vi "Power Qualtiy - 4.vi"() -> ()   [LabVIEW 2015]
uses:
  <vilib>/addons/Electrical Power/Basic/Measurement/subVIs/basic_Power Value.ctl
  <vilib>/express/express signal manip/GetorSetDDTAttributes/Shared VIs/TimeType.ctl
  <vilib>/express/express signal manip/GetorSetDDTAttributes/Shared VIs/XDimension.ctl
  <vilib>/addons/Electrical Power/Basic/Measurement/RMS (N Channels).vi
  <vilib>/addons/Electrical Power/Basic/Measurement/Power (1 Channel).vi
  <vilib>/express/express signal manip/GetorSetDDTAttributes/Shared VIs/TimeMode Enum to Boolean.vi
  <vilib>/express/express signal manip/GetorSetDDTAttributes/Shared VIs/XDimension Enum to String.vi
  <vilib>/express/express shared/transition.llb/Dynamic To Waveform Array.vi
  <vilib>/express/express signal manip/GetorSetDDTAttributes/Set DDT Attributes/SetT0.vi
  <vilib>/express/express signal manip/GetorSetDDTAttributes/Set DDT Attributes/sub Set StartTimeStamp.vi
  <vilib>/express/express shared/transition.llb/Waveform Array To Dynamic.vi
  <vilib>/express/express signal manip/GetorSetDDTAttributes/Set DDT Attributes/Set DDT Properties.xnode
  <vilib>/express/express signal manip/GetorSetDDTAttributes/Shared VIs/GetSetShared.lvlib
  <vilib>/addons/Electrical Power/Basic/NI_EP_Basic.lvlib
  <vilib>/express/express signal manip/GetorSetDDTAttributes/Set DDT Attributes/Set DDT Attributes.lvlib
panel:
  out "Voltage":dbl(knob) scale=0.0..230.0
  out "power value":T1
  out "Voltage Waveform":dynamicdata(graph)
  out "Current Waveform":dynamicdata(graph)
  out "Current":dbl(knob) scale=0.0..12.0
  out "THD":dbl
  out "Current Harmonics":dynamicdata(graph)
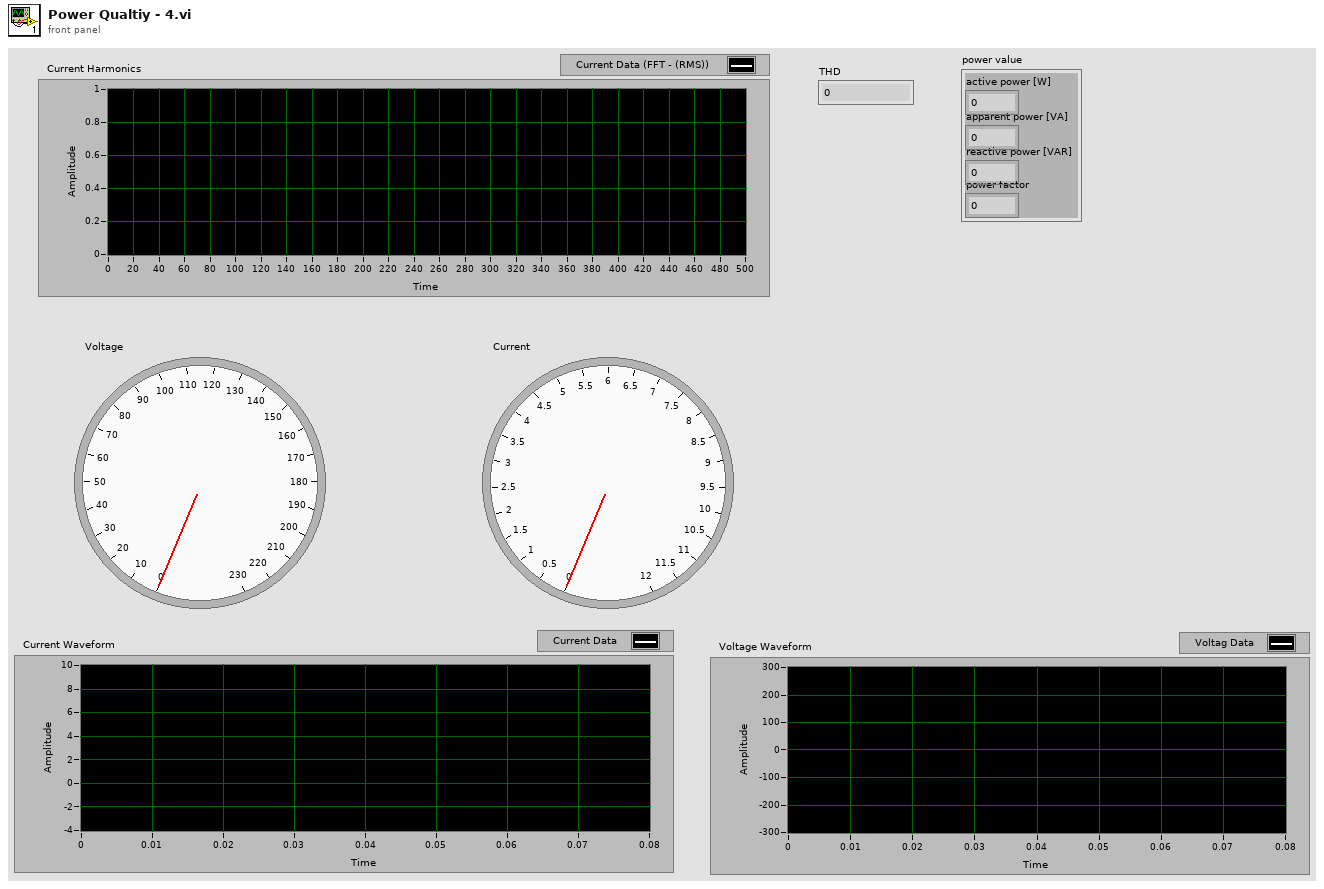
[diagram p1: front panel]
types:
  T1 = typedef "NI_EP_Basic.lvlib/basic_Power Value.ctl" = cluster{"active power [W]":dbl, "apparent power [VA]":dbl, "reactive power [VAR]":dbl, "power factor":dbl}
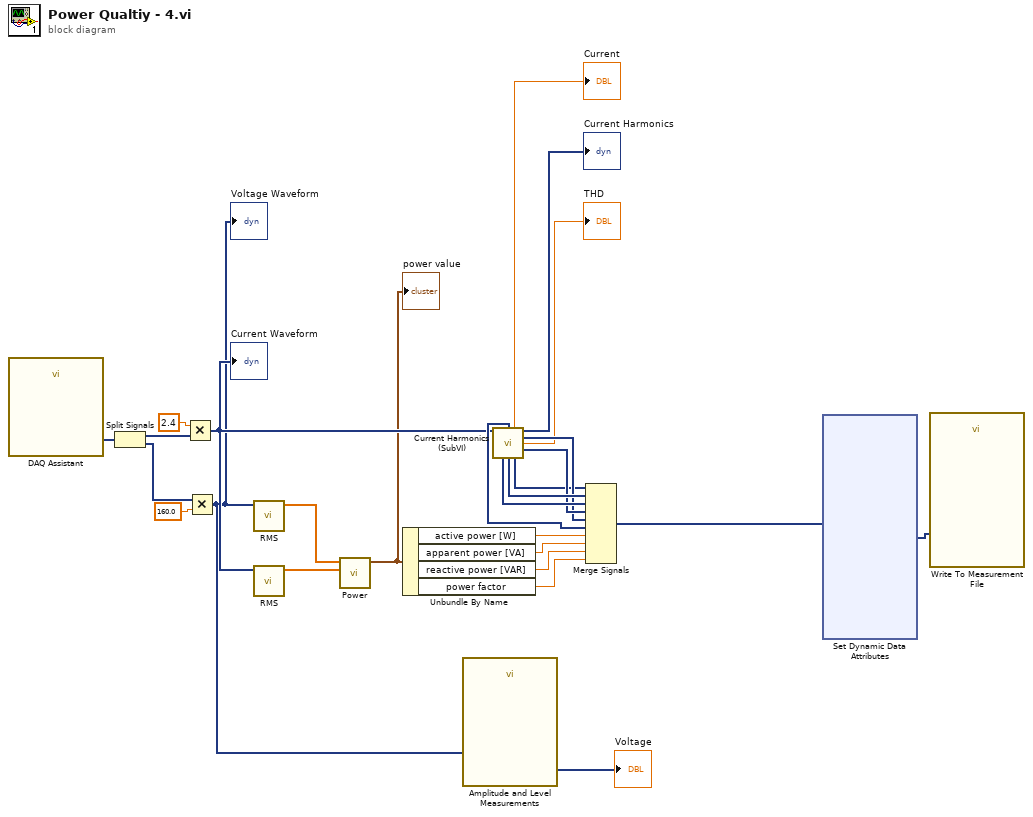
[diagram p0: block diagram]
diagram:
  n1 = call "DAQ Assistant"() -> ("data"=w26:dynamicdata)  [unwired: 17 in, 2 out]
  n2 = Split Signals(w26) -> (w25:dynamicdata, w24:dynamicdata)  [unwired: 2 in]
  n3 = Multiply(x=2.4, y=w25) -> (x*y=w10:dynamicdata)
  "Current Waveform" <- w10
  n4 = Multiply(x=w24, y=160.0) -> (x*y=w2:dynamicdata)
  "Voltage Waveform" <- w2
  n5 = call-poly <vilib>:"RMS.vi"("waveforms"=w2) -> ("RMS values"=w9:dbl[])  [unwired: 9 in, 1 out]
  n6 = call-poly <vilib>:"RMS.vi"("waveforms"=w10) -> ("RMS values"=w8:dbl[])  [unwired: 9 in, 1 out]
  n7 = call-poly <vilib>:"Power.vi"("current waveform"=w8, "voltage waveform"=w9) -> ("power value"=w7:T1)  [unwired: 8 in, 1 out]
  "power value" <- w7
  n8 = Unbundle By Name(w7) -> ("active power [W]"=w6:dbl, "apparent power [VA]"=w5:dbl, "reactive power [VAR]"=w4:dbl, "power factor"=w3:dbl)
  n9 = call "Amplitude and Level Measurements"("Signals"=w2) -> ("RMS"=→"Voltage":dynamicdata)  [unwired: 13 in, 1 out]
  n10 = call "Current Harmonics (SubVI).vi"("Dynamic Data"=w10) -> ("Specific Harmonic"=w17:dynamicdata, "Current"=→"Current":dbl, "Current Harmonics"=→"Current Harmonics":dynamicdata, "Specific Harmonic 2"=w18:dynamicdata, "THD"=→"THD":dbl, "Specific Harmonic 3"=w19:dynamicdata, "Specific Harmonic 4"=w20:dynamicdata, "THD 2"=w21:dynamicdata, "RMS"=w14:dynamicdata)  [unwired: 6 in]
  n11 = Merge Signals(w14, w21, w20, w19, w18, w17, w6, w5, w4, w3) -> (w16:dynamicdata)
  n12 = xnode "Set Dynamic Data Attributes"("Signals In"=w16) -> ("Signals Out"=w15:dynamicdata)  [unwired: 6 in, 1 out]
  n13 = call "Write To Measurement File"("Signals"=w15) -> ()  [unwired: 16 in, 3 out]
